vi "GraphAndChartsForThermresistorMarcoGonzalez.vi"() -> ()   [LabVIEW 2012]
panel:
  in  "stop":bool
  out "Multiple Graph":dbl[][](graph)
  out "Single Chart":dbl(graph)
  out "Single Graph":dbl[](graph)
  out "Multiple Chart":T1(graph)
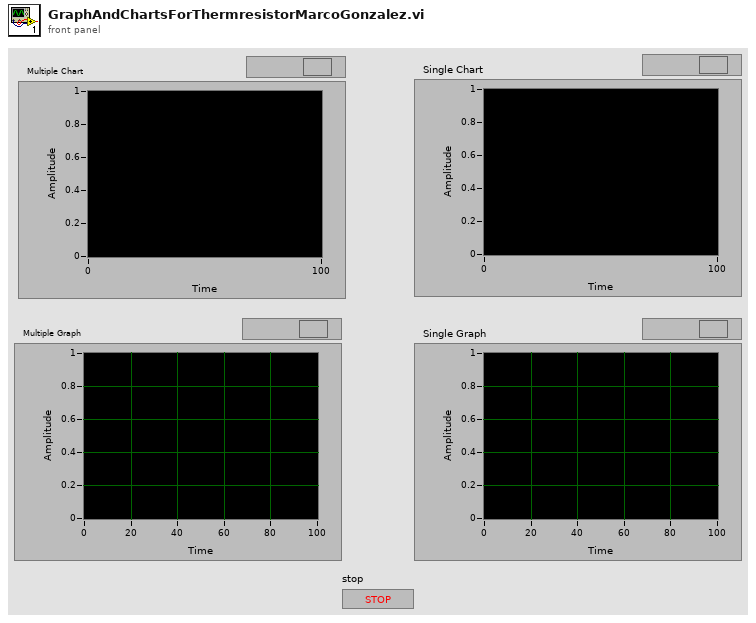
[diagram p1: front panel]
types:
  T1 = cluster{"number: 0 to 1":dbl, "number: 0 to 1":dbl}
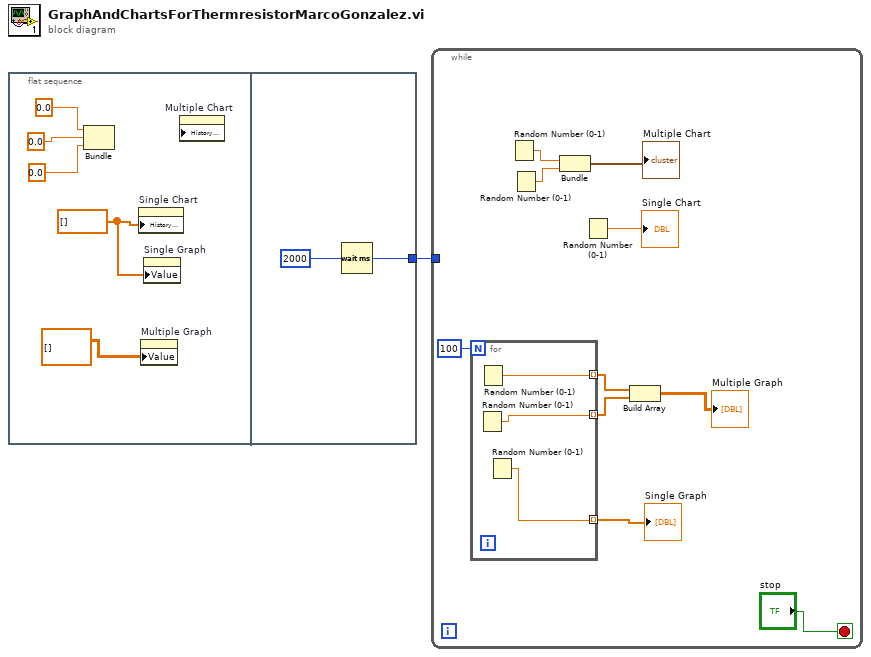
[diagram p0: block diagram]
diagram:
  n1 = flat-sequence {
    tunnel: [w7] -> w1
    frame #0 {
      w6 = dbl[] [] ("History Data")
      n2 = Bundle("element"=0.0, "element"=0.0, "element"=0.0) -> ()  [unwired: 1 in, 1 out]
      n3 = property on="Single Chart" class="WFChart (strict)"("History Data"=w6) -> ()  [unwired: 2 in, 2 out]
      n4 = property on="Multiple Graph" class="WFGraph (strict)"("Value"=dbl[][] []) -> ()  [unwired: 2 in, 2 out]
      n5 = property on="Single Graph" class="WFGraph (strict)"("Value"=w6) -> ()  [unwired: 2 in, 2 out]
      n6 = property on="Multiple Chart" class="WFChart (strict)" props=["History Data"]() -> ()  [unwired: 3 in, 2 out]
    }
    frame #1 {
      n7 = Wait (ms)(milliseconds to wait=u32 2000) -> (millisecond timer value=w7:u32)
    }
  }
  n8 = while {
    tunnel: w1 -> [_]
    stop <- "stop" stop-if-true
    n9 = for {
      N: 100 -> [_]
      tunnel: [w21] -> w13 mode=indexing
      tunnel: [w20] -> w11 mode=indexing
      tunnel: [w19] -> w12 mode=indexing
      n10 = Random Number (0-1)() -> (number: 0 to 1=w20:dbl)
      n11 = Random Number (0-1)() -> (number: 0 to 1=w19:dbl)
      n12 = Random Number (0-1)() -> (number: 0 to 1=w21:dbl)
    }
    "Single Graph" <- w13
    n13 = Random Number (0-1)() -> (number: 0 to 1=w18:dbl)
    n14 = Random Number (0-1)() -> (number: 0 to 1=w17:dbl)
    n15 = Bundle("number: 0 to 1"=w18, "number: 0 to 1"=w17) -> (→"Multiple Chart":T1)  [unwired: 1 in]
    n16 = Random Number (0-1)() -> (number: 0 to 1=→"Single Chart":dbl)
    n17 = Build Array(w12, w11) -> (→"Multiple Graph":dbl[][])
  }
